vi "DTACQ - Set AWG Length.vi"(8 "error in":errorcluster, 10 "AWG Length":i32, 11 "Address":string) -> (0 "error out":errorcluster)   [LabVIEW 2017, in "Communications Library.lvlib"]
doc: "Querries the status of the DTACQ device.\n\nThe status of both the module carrier and the analog out module are querried."
uses:
  Communications Library.lvlib
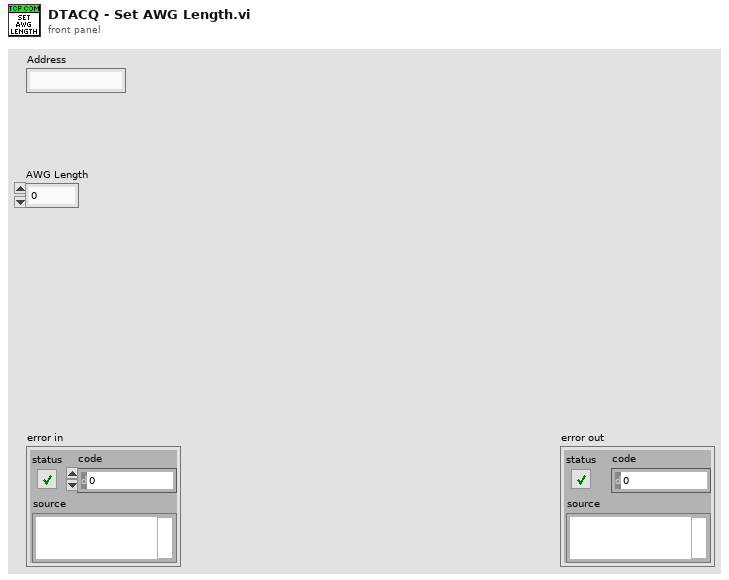
[diagram p1: front panel]
types:
  T1 = typedef "Communications Library.lvlib/DTACQ Connection Data--Cluster.ctl" = cluster{"Description":string, "Address":string, "Port":u16, "timeout (ms)":i32, "Termination Character":string, "TCP Connection Reference":refnum<k5>, "Open Connection":bool}
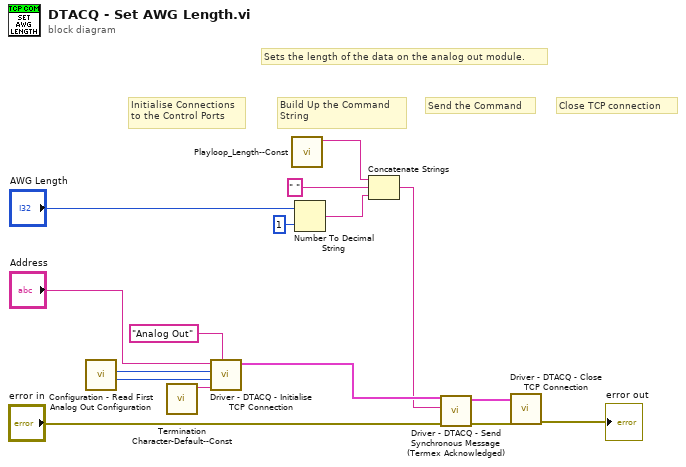
[diagram p0: block diagram]
diagram:
  # "Send the Command"
  # "Sets the length of the data on the analog out module."
  # "Close TCP connection"
  # "Build Up the Command\nString"
  # "Initialise Connections\nto the Control Ports"
  n1 = call "Configuration - Read First Analog Out Configuration.vi"() -> ("Timeout (ms)"=w11:i32, "Analog Out Control Port"=w12:i32)  [unwired: 7 in, 3 out]
  n2 = call "Termination Character-Default--Const.vi"() -> ("Termination Character"=w14:string)  [unwired: 11 in]
  n3 = call "Driver - DTACQ - Initialise TCP Connection.vi"("Description"="Analog Out", "Termination Character"=w14, "timeout (ms)"=w11, "Port"=w12, "Address"="Address") -> ("DTACQ Connection Data Out"=w9:T1)  [unwired: 6 in]
  n4 = call "Playloop_Length--Const.vi"() -> ("AWG Length Command"=w6:string)  [unwired: 11 in]
  n5 = Number To Decimal String(number="AWG Length", width (-)=i16 1) -> (decimal integer string=w3:string)
  n6 = Concatenate Strings(w6, " ", w3) -> (w1:string)
  n7 = call "Driver - DTACQ - Send Synchronous Message (Termex Acknowledged).vi"("error in"="error in", "Message to Send"=w1, "DTACQ Connection Data In"=w9) -> ("error out"=w7:errorcluster, "DTACQ Connection Data Out"=w8:T1)  [unwired: 5 in, 2 out]
  n8 = call "Driver - DTACQ - Close TCP Connection.vi"("error in"=w7, "DTACQ Connection Data In"=w8) -> ("error out"=→"error out":errorcluster)  [unwired: 8 in, 1 out]
